vi "main_ai.vi"() -> ()   [LabVIEW 2023]
uses:
  <vilib>/sound2/lvsound2.llb/Sound Output Set Volume (Single).vi
panel:
  in  "Reset":bool
  out "p2 score":i32
  out "p1 score":i32
  in  "Ball Speed":dbl(slide)=2.0 scale=0.0..5.0
  in  "Player Length":i32(slide)=100 scale=50.0..150.0
  in  "Pause Game":bool
  in  "Stop":bool
  in  "w_bool":bool
  in  "Down_bool":bool
  in  "s_bool":bool
  in  "Up_bool":bool
  out "game window":picture
  # "Player 1: W, S\nPlayer 2: Up, Down"
  # "Modifiers"
  # "Spacebar"
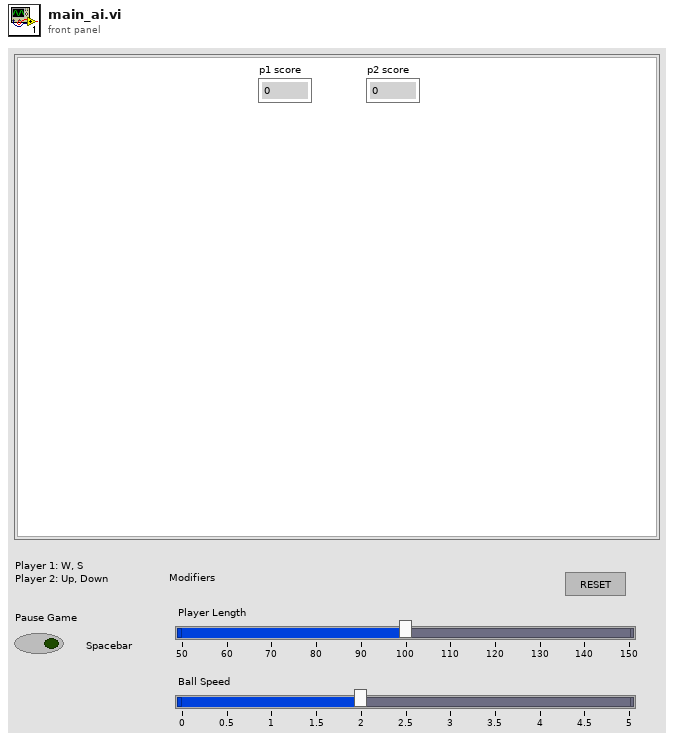
[diagram p1: front panel]
types:
  T1 = typedef "Sound Output Task ID.ctl" = u32
  T2 = cluster{"output vector x":dbl, "output vector y":dbl}
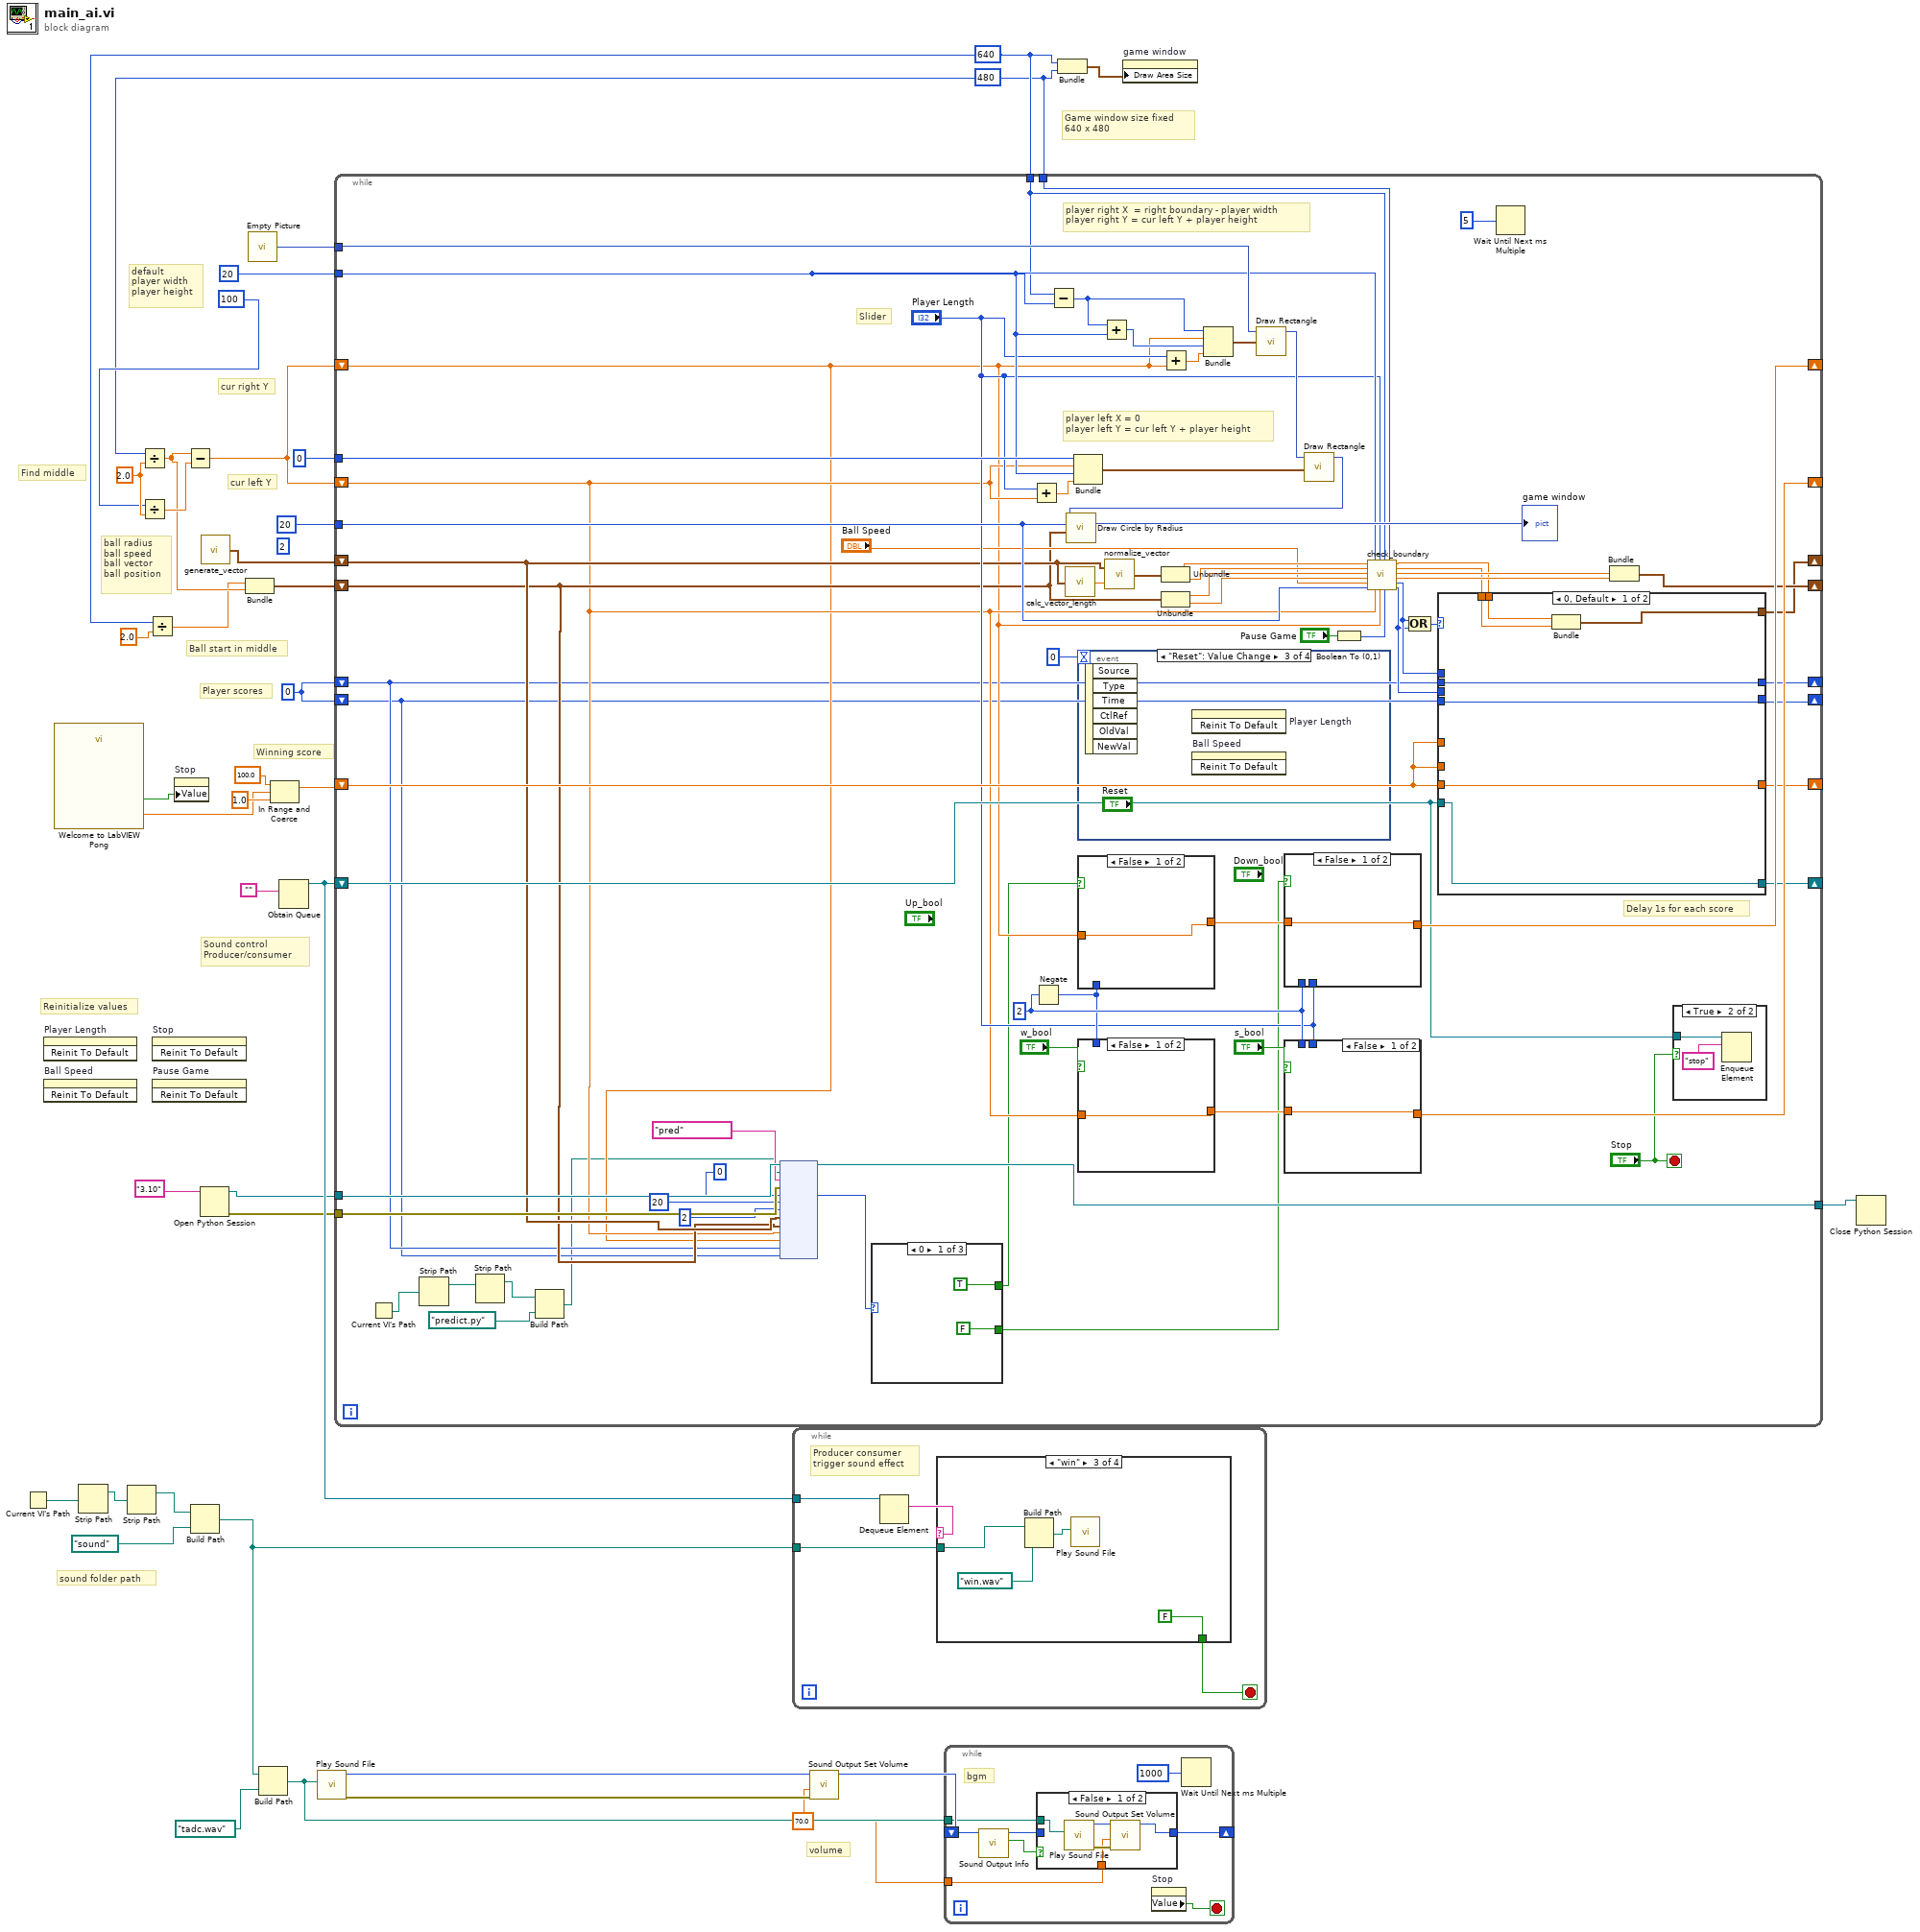
[diagram p0: block diagram]
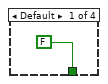
[diagram p3: hidden frame]
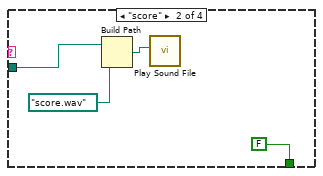
[diagram p4: hidden frame]
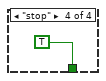
[diagram p5: hidden frame]
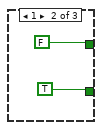
[diagram p6: hidden frame]
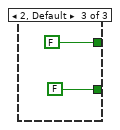
[diagram p7: hidden frame]
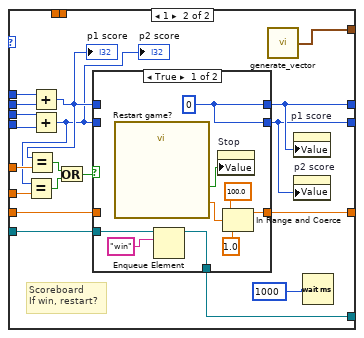
[diagram p9: hidden frame]
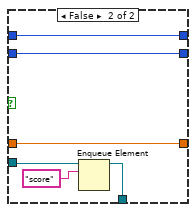
[diagram p10: hidden frame]
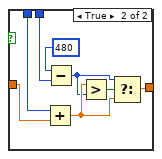
[diagram p11: hidden frame]
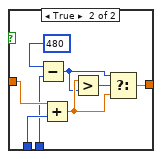
[diagram p12: hidden frame]
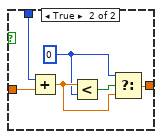
[diagram p13: hidden frame]
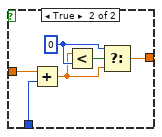
[diagram p14: hidden frame]
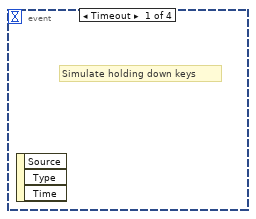
[diagram p15: hidden frame]
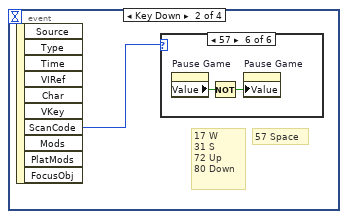
[diagram p16: hidden frame]
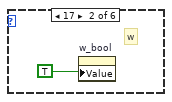
[diagram p18: hidden frame]
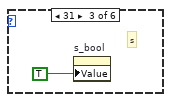
[diagram p19: hidden frame]
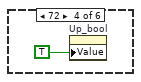
[diagram p20: hidden frame]
diagram:
  w6 = 70.0 ("volume")
  w24 = 0
  (unwired) 2
  w25 = 480
  w31 = 640
  w34 = 2.0 ("y")
  # "Reinitialize values"
  # "volume"
  # "sound folder path"
  # "Sound control\nProducer/consumer"
  # "Winning score"
  # "Player scores"
  # "Ball start in middle"
  # "ball radius\nball speed\nball vector\nball position"
  # "Find middle"
  # "default\nplayer width\nplayer height"
  # "cur left Y"
  # "cur right Y"
  # "Game window size fixed\n640 x 480"
  n1 = Current VI's Path() -> (path=w15:path)
  n2 = invoke on="Player Length" class="Slide (strict)" method="Reinit To Default"() -> ()  [unwired: 3 in, 3 out]
  n3 = invoke on="Ball Speed" class="Slide (strict)" method="Reinit To Default"() -> ()  [unwired: 3 in, 3 out]
  n4 = call "Welcome to LabVIEW Pong"() -> ("Winning Score"=w20:dbl, "Quit Game"=w5:bool)  [unwired: 17 in, 1 out]
  n5 = Strip Path(path=w15) -> (stripped path=w14:path)  [unwired: 1 out]
  n6 = Strip Path(path=w14) -> (stripped path=w16:path)  [unwired: 1 out]
  n7 = Divide(x=w25, y=w34) -> (x/y=w28:dbl)
  n8 = Divide(x=100, y=w34) -> (x/y=w33:dbl)
  n9 = Divide(x=w31, y=2.0) -> (x/y=w27:dbl)
  n10 = invoke on="Stop" class="Bool (strict)" method="Reinit To Default"() -> ()  [unwired: 3 in, 3 out]
  n11 = invoke on="Pause Game" class="Bool (strict)" method="Reinit To Default"() -> ()  [unwired: 3 in, 3 out]
  n12 = property on="Stop" class="Bool (strict)"("Value"=w5) -> ()  [unwired: 2 in, 2 out]
  n13 = Subtract(x=w28, y=w33) -> (x-y=w35:dbl)
  n14 = Build Path(base path=w16, name or relative path=path "sound") -> (appended path=w12:path)
  n15 = Open Python Session(python version="3.10" ("Python version")) -> (session out=w4:refnum<k35>, error out=w2:errorcluster)  [unwired: 2 in]
  n16 = call "generate_vector.vi"() -> ("Cluster"=w23:cluster{"number":dbl, "number":dbl})
  n17 = Bundle(w27, w28) -> (w29:cluster{dbl, dbl})  [unwired: 1 in]
  n18 = call "Empty Picture"() -> ("empty picture"=w38:picture)
  n19 = Build Path(base path=w12, name or relative path=path "tadc.wav") -> (appended path=w10:path)
  n20 = In Range and Coerce(upper limit=100.0, x=w20, lower limit=1.0) -> (coerced(x)=w21:dbl)  [unwired: 1 out]
  n21 = Obtain Queue(element data type="") -> (queue out=w11:refnum<queue>)  [unwired: 4 in, 2 out]
  n22 = call <vilib>:"Play Sound File.vi"("path"=w10) -> ("error out"=w8:errorcluster, "task ID"=w9:T1)  [unwired: 9 in]
  n23 = while {
    tunnel: w31 -> [w83]
    tunnel: w38 -> [w108]
    shift-right: [w97] -> _
    shift-left: w35 -> [w50]
    shift-right: [w95] -> _
    shift-left: w35 -> [w51]
    tunnel: 20 -> [w84]
    tunnel: 0 -> [w106]
    shift-right: [w72] -> _
    shift-left: w23 -> [w53]
    shift-right: [w79] -> _
    shift-left: w29 -> [w52]
    tunnel: 20 -> [w78]
    tunnel: w25 -> [w82]
    shift-right: [w77] -> _
    shift-left: w24 -> [w49]
    shift-right: [w76] -> _
    shift-left: w24 -> [w48]
    shift-right: [w75] -> _
    shift-left: w21 -> [w71]
    shift-right: [w65] -> _
    shift-left: w11 -> [w63]
    tunnel: w4 -> [w60]
    tunnel: [w59] -> w3
    tunnel: w2 -> [w58]
    stop <- "Stop" stop-if-true
    w100 = 2 ("y")
    # "Slider"
    # "Delay 1s for each score"
    # "player right X  = right boundary - player width\nplayer right Y = cur left Y + player height"
    # "player left X = 0\nplayer left Y = cur left Y + player height"
    n24 = Current VI's Path() -> (path=w44:path)
    n25 = Strip Path(path=w44) -> (stripped path=w43:path)  [unwired: 1 out]
    n26 = Strip Path(path=w43) -> (stripped path=w42:path)  [unwired: 1 out]
    n27 = Build Path(base path=w42, name or relative path=path "predict.py") -> (appended path=w40:path)
    n28 = node(w60, w40, "pred" ("function name"), w58, 0, 20, 2, w53, w52, w51, w50, w49, w48) -> (w59:refnum<k35>, w47:i32)  [unwired: 8 in, 3 out]
    n29 = case shown="0" w47 {
      tunnel: [TRUE FALSE FALSE] -> w46
      tunnel: [FALSE TRUE FALSE] -> w45
      frame 0 {
      }
      frame 1 {
      }
      frame 2, Default {
      }
    }
    n30 = Add(x="Player Length", y=w51) -> (x+y=w105:dbl)
    n31 = Negate(x=w100) -> (-x=w99:i32)
    n32 = Subtract(x=w83, y=w84) -> (x-y=w111:i32)
    n33 = call "calc_vector_length.vi"("vector"=w53) -> ("length"=w89:dbl)
    n34 = Bundle(w106, w51, w84, w105) -> (w104:cluster{i32, dbl, i32, dbl})  [unwired: 1 in]
    n35 = event shown="[2] \"Reset\": Value Change" {
      selector: _ -> [_ _ _ _]
      dyn-events: _ -> [_ _ _ _]
      timeout: 0 -> [_ _ _ _]
      event Timeout {
        # "Simulate holding down keys"
        n36 = event-data() -> ()  [unwired: 1 in, 3 out]
      }
      event Key Down {
        # "57 Space"
        # "17 W\n31 S\n72 Up\n80 Down"
        n37 = event-data() -> ("ScanCode"=w193:i16)  [unwired: 1 in, 9 out]
        n38 = case shown="57" w193 {
          frame 0, Default {
          }
          frame 17 {
            # "w"
            n39 = property on="w_bool" class="Bool (strict)"("Value"=TRUE) -> ()  [unwired: 2 in, 2 out]
          }
          frame 31 {
            # "s"
            n40 = property on="s_bool" class="Bool (strict)"("Value"=TRUE) -> ()  [unwired: 2 in, 2 out]
          }
          frame 72 {
            n41 = property on="Up_bool" class="Bool (strict)"("Value"=TRUE) -> ()  [unwired: 2 in, 2 out]
          }
          frame 80 {
            n42 = property on="Down_bool" class="Bool (strict)"("Value"=TRUE) -> ()  [unwired: 2 in, 2 out]
          }
          frame 57 {
            n43 = property on="Pause Game" class="Bool (strict)"() -> ("Value"=w198:bool)  [unwired: 2 in, 2 out]
            n44 = Not(x=w198) -> (.not. x?=w199:bool)
            n45 = property on="Pause Game" class="Bool (strict)"("Value"=w199) -> ()  [unwired: 2 in, 2 out]
          }
        }
      }
      event "Reset": Value Change {
        n46 = event-data() -> ()  [unwired: 1 in, 6 out]
        n47 = invoke on="Player Length" class="Slide (strict)" method="Reinit To Default"() -> ()  [unwired: 3 in, 3 out]
        n48 = invoke on="Ball Speed" class="Slide (strict)" method="Reinit To Default"() -> ()  [unwired: 3 in, 3 out]
      }
      event Key Up {
        n49 = event-data() -> ("ScanCode"=w200:i16)  [unwired: 1 in, 5 out]
        n50 = case shown="72" w200 {
          frame 0, Default {
          }
          frame 17 {
            # "w"
            n51 = property on="w_bool" class="Bool (strict)"("Value"=FALSE) -> ()  [unwired: 2 in, 2 out]
          }
          frame 31 {
            # "s"
            n52 = property on="s_bool" class="Bool (strict)"("Value"=FALSE) -> ()  [unwired: 2 in, 2 out]
          }
          frame 72 {
            n53 = property on="Up_bool" class="Bool (strict)"("Value"=FALSE) -> ()  [unwired: 2 in, 2 out]
          }
          frame 80 {
            n54 = property on="Down_bool" class="Bool (strict)"("Value"=FALSE) -> ()  [unwired: 2 in, 2 out]
          }
        }
      }
    }
    n55 = case shown="False" w46 {
      tunnel: w99 -> [_ w188]
      tunnel: w50 -> [w186 w189]
      tunnel: [w186 w187] -> w98
      frame False {
      }
      frame True {
        w191 = 0 ("y")
        n56 = Add(x=w189, y=w188) -> (x+y=w190:dbl)
        n57 = Less?(x=w190, y=w191) -> (x < y?=w192:bool)
        n58 = Select(t=w191, s=w192, f=w190) -> (s? t:f=w187:dbl)
      }
    }
    n59 = case shown="False" "w_bool" {
      tunnel: w51 -> [w179 w181]
      tunnel: w99 -> [_ w182]
      tunnel: [w179 w180] -> w96
      frame False {
      }
      frame True {
        w183 = 0 ("y")
        n60 = Add(x=w182, y=w181) -> (x+y=w185:dbl)
        n61 = Less?(x=w185, y=w183) -> (x < y?=w184:bool)
        n62 = Select(t=w183, s=w184, f=w185) -> (s? t:f=w180:dbl)
      }
    }
    n63 = Add(x=w111, y=w84) -> (x+y=w110:i32)
    n64 = call "normalize_vector.vi"("Numeric"=w89, "vector"=w53) -> ("output"=w90:cluster{"x":dbl, "y":dbl})
    n65 = Unbundle(w90) -> ("x"=w88:dbl, "y"=w87:dbl)
    n66 = Unbundle(w52) -> (w86:dbl, w85:dbl)
    n67 = Add(x="Player Length", y=w50) -> (x+y=w109:dbl)
    n68 = Bundle(w111, w50, w110, w109) -> (w107:cluster{i32, dbl, i32, dbl})  [unwired: 1 in]
    n69 = call <vilib>:"Draw Rectangle.vi"("picture"=w108, "rect"=w107) -> ("new picture"=w103:picture)  [unwired: 7 in]
    n70 = case shown="False" w45 {
      tunnel: w100 -> [_ w174]
      tunnel: w98 -> [w170 w173]
      tunnel: [w170 w172] -> w97
      tunnel: "Player Length" -> [_ w171]
      frame False {
      }
      frame True {
        n71 = Subtract(x=480 ("y"), y=w171) -> (x-y=w176:i32)
        n72 = Add(x=w173, y=w174) -> (x+y=w177:dbl)
        n73 = Greater?(x=w177, y=w176) -> (0:w178:bool)
        n74 = Select(t=w176, s=w178, f=w177) -> (s? t:f=w172:dbl)
      }
    }
    n75 = case shown="False" "s_bool" {
      tunnel: w100 -> [_ w164]
      tunnel: w96 -> [w161 w165]
      tunnel: [w161 w163] -> w95
      tunnel: "Player Length" -> [_ w162]
      frame False {
      }
      frame True {
        n76 = Add(x=w164, y=w165) -> (x+y=w168:dbl)
        n77 = Subtract(x=480 ("y"), y=w162) -> (x-y=w167:i32)
        n78 = Greater?(x=w168, y=w167) -> (0:w169:bool)
        n79 = Select(t=w167, s=w169, f=w168) -> (s? t:f=w163:dbl)
      }
    }
    n80 = call <vilib>:"Draw Rectangle.vi"("picture"=w103, "rect"=w104) -> ("new picture"=w92:picture)  [unwired: 7 in]
    n81 = call <vilib>:"Draw Circle by Radius.vi"("pixel center"=w52, "radius"=w78, "picture"=w92) -> ("new picture"=→"game window":picture)  [unwired: 8 in]
    n82 = Boolean To (0,1)(Boolean="Pause Game") -> (0, 1=w66:i16)
    n83 = call "check_boundary.vi"("vector x"=w88, "vector y"=w87, "position x"=w86, "position y"=w85, "speed"="Ball Speed", "radius"=w78, "player width"=w84, "player left position y"=w51, "player height"="Player Length", "player right position y"=w50, "window width"=w83, "pause"=w66, "window height"=w82) -> ("output vector x"=w74:dbl, "output vector y"=w73:dbl, "output x"=w81:dbl, "output y"=w80:dbl, "left win"=w69:i32, "right win"=w68:i32)  [unwired: 1 in]
    n84 = Compound Arithmetic op=OR(w69, w68) -> (w70:i32)
    n85 = case shown="0, Default" w70 {
      tunnel: w49 -> [w126 w136]
      tunnel: w48 -> [w125 w134]
      tunnel: w69 -> [_ w137]
      tunnel: w68 -> [_ w135]
      tunnel: [w126 w130] -> w77
      tunnel: [w125 w129] -> w76
      tunnel: w71 -> [_ w145]
      tunnel: w71 -> [_ w144]
      tunnel: [w124 w140] -> w75
      tunnel: w71 -> [w124 w139]
      tunnel: w74 -> [w123 _]
      tunnel: w73 -> [w122 _]
      tunnel: [w121 w138] -> w72
      tunnel: w63 -> [w120 w128]
      tunnel: [w120 w127] -> w65
      frame 0, Default {
        n86 = Bundle("output vector x"=w123, "output vector y"=w122) -> (w121:T2)  [unwired: 1 in]
      }
      frame 1 {
        # "Scoreboard\nIf win, restart?"
        n87 = Add(x=w137, y=w136) -> (x+y=w132:i32)
        "p1 score" <- w132
        n88 = Equal?(x=w132, y=w145) -> (x = y?=w142:bool)
        n89 = Add(x=w135, y=w134) -> (x+y=w131:i32)
        "p2 score" <- w131
        n90 = Equal?(x=w131, y=w144) -> (x = y?=w141:bool)
        n91 = Or(x=w142, y=w141) -> (x .or. y?=w143:bool)
        n92 = case shown="True" w143 {
          tunnel: [w153 w158] -> w129
          tunnel: [w153 w159] -> w130
          tunnel: [w150 w160] -> w140
          tunnel: w139 -> [_ w160]
          tunnel: w132 -> [_ w159]
          tunnel: w131 -> [_ w158]
          tunnel: w128 -> [w148 w156]
          tunnel: [w146 w155] -> w127
          frame True {
            w153 = 0
            n93 = call "Restart game?"() -> ("Winning Score"=w149:dbl, "Quit game"=w154:bool)  [unwired: 17 in, 1 out]
            n94 = Enqueue Element(queue=w148, element="win") -> (queue out=w146:refnum<queue>)  [unwired: 2 in, 2 out]
            n95 = property on="Stop" class="Bool (strict)"("Value"=w154) -> ()  [unwired: 2 in, 2 out]
            n96 = In Range and Coerce(upper limit=100.0, x=w149, lower limit=1.0) -> (coerced(x)=w150:dbl)  [unwired: 1 out]
          }
          frame False {
            n97 = Enqueue Element(queue=w156, element="score") -> (queue out=w155:refnum<queue>)  [unwired: 2 in, 2 out]
          }
        }
        n98 = call "generate_vector.vi"() -> ("Cluster"=w138:cluster{"number":dbl, "number":dbl})
        n99 = property on="p1 score" class="DigNum (strict)"("Value"=w130) -> ()  [unwired: 2 in, 2 out]
        n100 = property on="p2 score" class="DigNum (strict)"("Value"=w129) -> ()  [unwired: 2 in, 2 out]
        n101 = Wait (ms)(milliseconds to wait=u32 1000) -> ()  [unwired: 1 out]
      }
    }
    n102 = Wait Until Next ms Multiple(millisecond multiple=u32 5 ("milliseconds to wait")) -> ()  [unwired: 1 out]
    n103 = Bundle("output x"=w81, "output y"=w80) -> (w79:cluster{"output x":dbl, "output y":dbl})  [unwired: 1 in]
    n104 = case shown="True" "Stop" {
      tunnel: w63 -> [_ w119]
      frame False {
      }
      frame True {
        n105 = Enqueue Element(queue=w119, element="stop") -> ()  [unwired: 2 in, 3 out]
      }
    }
  }
  n106 = while {
    tunnel: w11 -> [w208]
    tunnel: w12 -> [w206]
    stop <- w205 stop-if-true
    # "Producer consumer\ntrigger sound effect"
    n107 = Dequeue Element(queue=w208) -> (element=w207:string)  [unwired: 2 in, 3 out]
    n108 = case shown="\"win\"" w207 {
      tunnel: w206 -> [_ w213 w217 _]
      tunnel: [FALSE ("Stop") FALSE ("Stop") FALSE ("Stop") TRUE ("Stop")] -> w205
      frame Default {
      }
      frame "score" {
        n109 = Build Path(base path=w213, name or relative path=path "score.wav") -> (appended path=w210:path)
        n110 = call <vilib>:"Play Sound File.vi"("path"=w210) -> ()  [unwired: 9 in, 2 out]
      }
      frame "win" {
        n111 = Build Path(base path=w217, name or relative path=path "win.wav") -> (appended path=w214:path)
        n112 = call <vilib>:"Play Sound File.vi"("path"=w214) -> ()  [unwired: 9 in, 2 out]
      }
      frame "stop" {
      }
    }
  }
  n113 = call-poly <vilib>:"Sound Output Set Volume.vi"("error in (no error)"=w8, "volume"=w6, "task ID"=w9) -> ("task ID out"=w7:T1)  [unwired: 7 in, 1 out]
  n114 = while {
    shift-right: [w222] -> _
    shift-left: w7 -> [w224]
    tunnel: w10 -> [w220]
    tunnel: w6 -> [w219]
    stop <- w225 stop-if-true
    # "bgm"
    n115 = call <vilib>:"Sound Output Info.vi"("task ID"=w224) -> ("is playing?"=w223:bool, "task ID out"=w221:T1)  [unwired: 7 in, 2 out]
    n116 = case shown="False" w223 {
      tunnel: [w228 w232] -> w222
      tunnel: w221 -> [_ w232]
      tunnel: w220 -> [w231 _]
      tunnel: w219 -> [w227 _]
      frame False {
        n117 = call <vilib>:"Play Sound File.vi"("path"=w231) -> ("error out"=w230:errorcluster, "task ID"=w229:T1)  [unwired: 9 in]
        n118 = call-poly <vilib>:"Sound Output Set Volume.vi"("error in (no error)"=w230, "volume"=w227, "task ID"=w229) -> ("task ID out"=w228:T1)  [unwired: 7 in, 1 out]
      }
      frame True {
      }
    }
    n119 = property on="Stop" class="Bool (strict)"() -> ("Value"=w225:bool)  [unwired: 2 in, 2 out]
    n120 = Wait Until Next ms Multiple(millisecond multiple=u32 1000) -> ()  [unwired: 1 out]
  }
  n121 = Bundle(w31, w25) -> (w39:cluster{i32, i32})  [unwired: 1 in]
  n122 = property on="game window" class="Pict"("Draw Area Size"=w39) -> ()  [unwired: 2 in, 2 out]
  n123 = Close Python Session(session in=w3) -> ()  [unwired: 1 in, 1 out]
